vi "Control.vi"() -> ()   [LabVIEW 2020]
uses:
  proceso1.vi
  proceso2.vi
  proceso3.vi
  proceso4.vi
  proceso5.vi
  proceso6.vi
panel:
  in  "Numeric 14":dbl
  in  "Numeric 13":dbl
  in  "Numeric 12":dbl
  in  "Numeric 11":dbl
  in  "Numeric 10":dbl
  out "Boolean":bool
  in  "Numeric 9":dbl
  in  "Numeric 8":dbl
  in  "Numeric 7":dbl
  in  "Numeric 6":dbl
  in  "Numeric 5":dbl
  in  "Numeric 4":dbl
  in  "Numeric 3":dbl
  in  "Numeric 2":dbl
  out "s? t:f":dbl
  in  "Numeric":dbl
types:
  T1 = typedef "Semaphore RefNum" = refnum<k1>
  T2 = cluster{"final_linea":bool, "vent 1":bool, "vent 2":bool, "vent 3":bool, "mov caja 2 horizontal":i32, "llenado caja 2":u8, "pos_inicial_horizontal":dbl, " pos_final_horizontal":dbl, "contador":dbl, "mov caja 2  vertical":i32, "pos_inicial_vertical":dbl, " pos_final_vertical":dbl}
  T3 = cluster{"sensor_refrigerador":bool, "temperatura":dbl, "tuberia 5":u8, "tuberia 6":u8}
  T4 = cluster{"sensor_intercambiador":bool, "sensor_caldera":bool, "sensor_bomba_2 ":bool, "tuberia 2":u8, "tuberia 3":u8, "tuberia 4":u8, "temperatura":dbl}
  T5 = cluster{"sensor_bomba_1":bool, "tanque in":u8, " tuberia 1":u8}
  T6 = cluster{"sensor_caja":bool, "vent 1":bool, "vent 2":bool, "vent 3":bool, "pos_inicial":dbl, "pos_final":dbl, "mov_caja 1":i32}
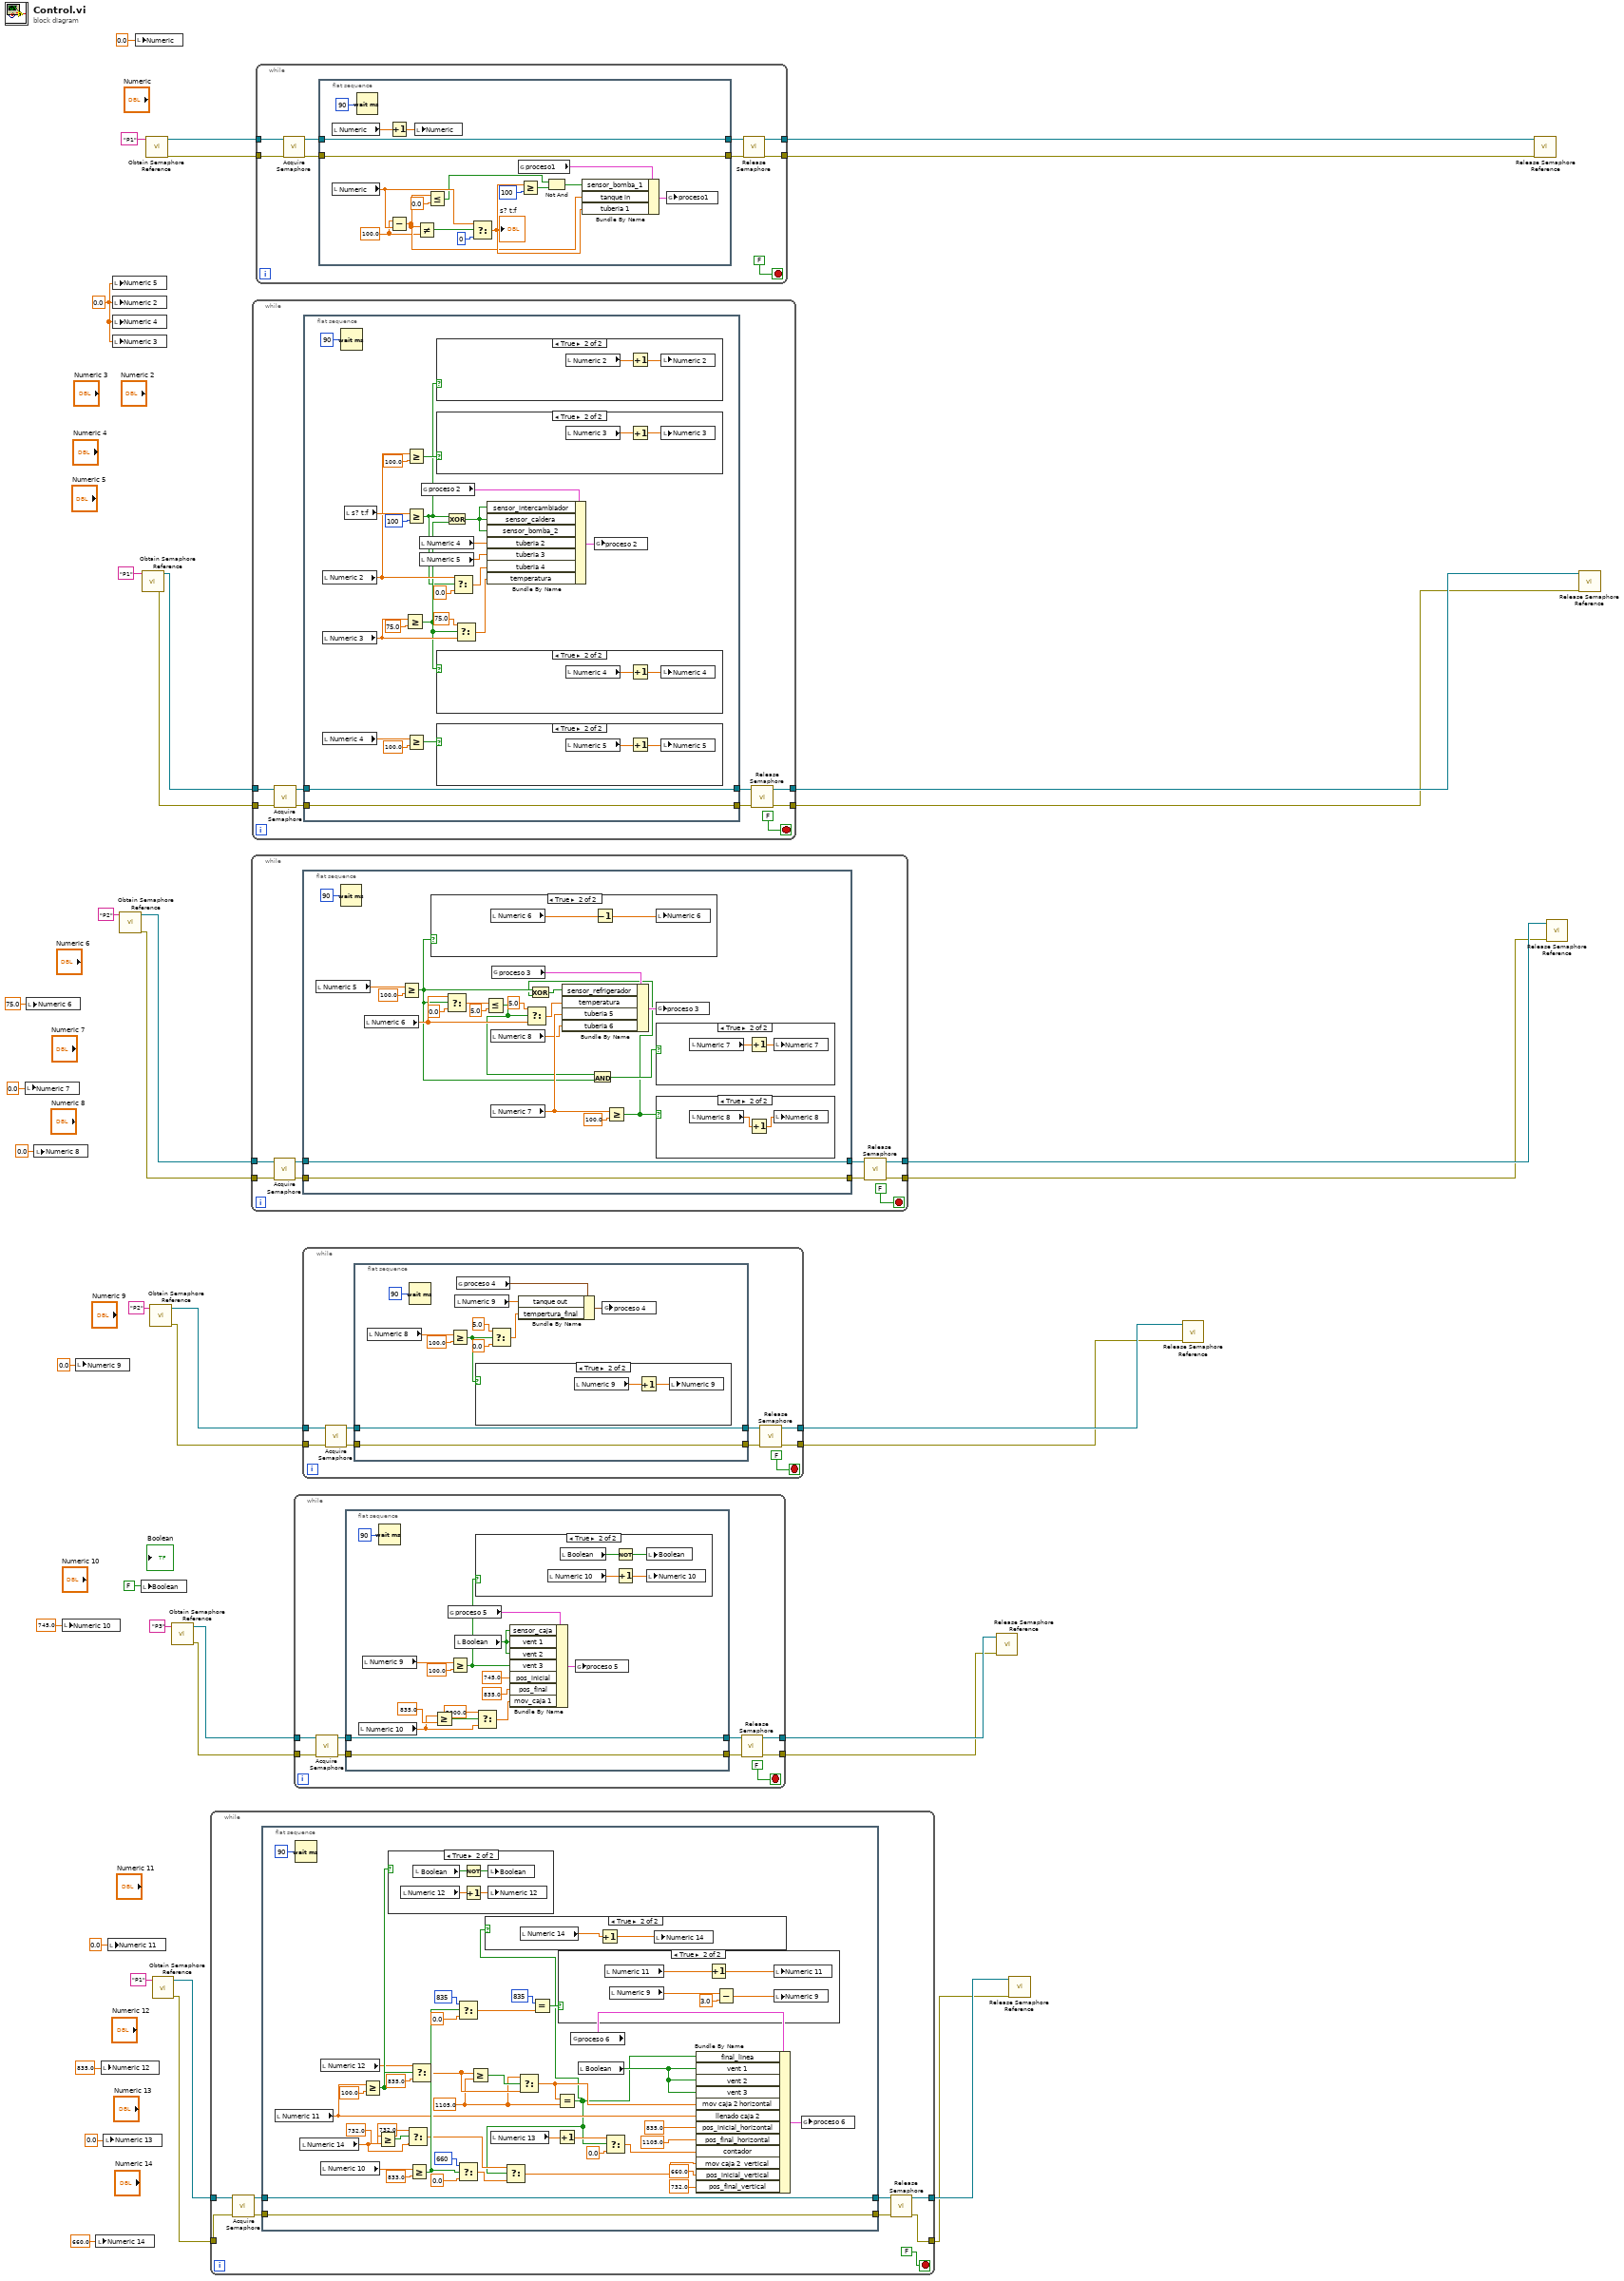
[diagram p0: block diagram]
diagram:
  w31 = 0.0 ("Numeric 2")
  n1 = local write "Numeric 7"(0.0 ("Numeric 7")) -> ()
  n2 = local write "Numeric 6"(75.0 ("Numeric 6")) -> ()
  n3 = local write "Numeric 8"(0.0 ("Numeric 8")) -> ()
  n4 = local write "Numeric 10"(745.0 ("Numeric 10")) -> ()
  n5 = local write "Numeric 9"(0.0 ("Numeric 9")) -> ()
  n6 = local write "Numeric 14"(660.0 ("Numeric 14")) -> ()
  n7 = local write "Numeric 12"(835.0 ("Numeric 12")) -> ()
  n8 = local write "Numeric 13"(0.0 ("Numeric 13")) -> ()
  n9 = local write "Numeric 11"(0.0 ("Numeric 11")) -> ()
  n10 = local write "Numeric 5"(w31) -> ()
  n11 = local write "Numeric 2"(w31) -> ()
  n12 = local write "Numeric 4"(w31) -> ()
  n13 = local write "Numeric 3"(w31) -> ()
  n14 = call <vilib>:"Obtain Semaphore Reference.vi"("name (unnamed)"="P2") -> ("error out"=w29:errorcluster, "semaphore"=w30:T1)  [unwired: 4 in, 1 out]
  n15 = local write "Numeric"(0.0 ("Numeric")) -> ()
  n16 = local write "Boolean"(FALSE ("Boolean")) -> ()
  n17 = call <vilib>:"Obtain Semaphore Reference.vi"("name (unnamed)"="P1") -> ("error out"=w33:errorcluster, "semaphore"=w32:T1)  [unwired: 4 in, 1 out]
  n18 = call <vilib>:"Obtain Semaphore Reference.vi"("name (unnamed)"="P1") -> ("error out"=w35:errorcluster, "semaphore"=w34:T1)  [unwired: 4 in, 1 out]
  n19 = call <vilib>:"Obtain Semaphore Reference.vi"("name (unnamed)"="P2") -> ("error out"=w21:errorcluster, "semaphore"=w22:T1)  [unwired: 4 in, 1 out]
  n20 = call <vilib>:"Obtain Semaphore Reference.vi"("name (unnamed)"="P1") -> ("error out"=w9:errorcluster, "semaphore"=w10:T1)  [unwired: 4 in, 1 out]
  n21 = call <vilib>:"Obtain Semaphore Reference.vi"("name (unnamed)"="P3") -> ("error out"=w16:errorcluster, "semaphore"=w17:T1)  [unwired: 4 in, 1 out]
  n22 = while {
    tunnel: w10 -> [w50]
    tunnel: w9 -> [w49]
    tunnel: [w44] -> w8
    tunnel: [w43] -> w7
    stop <- FALSE stop-if-true
    n23 = call <vilib>:"Acquire Semaphore.vi"("error in (no error)"=w49, "semaphore"=w50) -> ("error out"=w46:errorcluster, "semaphore out"=w48:T1)  [unwired: 3 in, 1 out]
    n24 = flat-sequence {
      tunnel: w48 -> [w81]
      tunnel: [w81] -> w47
      tunnel: w46 -> [w89]
      tunnel: [w89] -> w45
      frame #0 {
        w64 = 1105.0 ("y")
        n25 = local read "Numeric 11"() -> (w73:dbl)
        n26 = Wait (ms)(milliseconds to wait=u32 90) -> ()  [unwired: 1 out]
        n27 = local read "Numeric 14"() -> (w56:dbl)
        n28 = local read "Numeric 12"() -> (w68:dbl)
        n29 = local read "Numeric 10"() -> (w86:dbl)
        n30 = Greater Or Equal?(x=w73, y=100.0) -> (x >= y?=w69:bool)
        n31 = Greater Or Equal?(x=w56, y=732.0) -> (x >= y?=w58:bool)
        n32 = case shown="True" w69 {
          frame False {
          }
          frame True {
            n33 = local read "Numeric 12"() -> (w98:dbl)
            n34 = local read "Boolean"() -> (w95:bool)
            n35 = Not(x=w95) -> (.not. x?=w96:bool)
            n36 = Increment(x=w98) -> (x+1=w97:dbl)
            n37 = local write "Boolean"(w96) -> ()
            n38 = local write "Numeric 12"(w97) -> ()
          }
        }
        n39 = Select(t=732.0, s=w58, f=w56) -> (s? t:f=w55:dbl)
        n40 = Greater Or Equal?(x=w86, y=833.0) -> (x >= y?=w83:bool)
        n41 = Select(t=w68, s=w69, f=835.0) -> (s? t:f=w66:dbl)
        n42 = Select(t=835 ("mov caja 2 horizontal"), s=w83, f=0.0) -> (s? t:f=w71:dbl)
        n43 = Select(t=660 ("mov caja 2  vertical"), s=w83, f=0.0) -> (s? t:f=w54:dbl)
        n44 = Greater Or Equal?(x=w66, y=w64) -> (x >= y?=w67:bool)
        n45 = local read "Numeric 13"() -> (w63:dbl)
        n46 = Select(t=w64, s=w67, f=w66) -> (s? t:f=w65:dbl)
        n47 = Equal?(x=835, y=w71) -> (x = y?=w75:bool)
        n48 = Equal?(x=w65, y=w64) -> (x = y?=w52:bool)
        n49 = case shown="True" w52 {
          frame False {
          }
          frame True {
            n50 = local read "Numeric 14"() -> (w93:dbl)
            n51 = Increment(x=w93) -> (x+1=w94:dbl)
            n52 = local write "Numeric 14"(w94) -> ()
          }
        }
        n53 = Select(t=w55, s=w52, f=w54) -> (s? t:f=w53:dbl)
        n54 = Increment(x=w63) -> (x+1=w62:dbl)
        n55 = case shown="True" w75 {
          frame False {
          }
          frame True {
            n56 = local read "Numeric 11"() -> (w103:dbl)
            n57 = local read "Numeric 9"() -> (w101:dbl)
            n58 = Increment(x=w103) -> (x+1=w102:dbl)
            n59 = Subtract(x=w101, y=3.0) -> (x-y=w100:dbl)
            n60 = local write "Numeric 11"(w102) -> ()
            n61 = local write "Numeric 9"(w100) -> ()
          }
        }
        n62 = global read "proceso6.vi" "proceso 6"() -> (w92:T2)
        n63 = local read "Boolean"() -> (w90:bool)
        n64 = Select(t=w62, s=w52, f=0.0) -> (s? t:f=w60:dbl)
        n65 = Bundle By Name(cluster=w92, "final_linea"=w52, "vent 1"=w90, "vent 2"=w90, "vent 3"=w90, "mov caja 2 horizontal"=w65, "llenado caja 2"=w73, "pos_inicial_horizontal"=835.0, "pos_final_horizontal"=1105.0, "contador"=w60, "mov caja 2  vertical"=w53, "pos_inicial_vertical"=660.0, "pos_final_vertical"=732.0) -> (w91:T2)
        n66 = global write "proceso6.vi" "proceso 6"(w91) -> ()
      }
    }
    n67 = call <vilib>:"Release Semaphore.vi"("error in (no error)"=w45, "semaphore"=w47) -> ("error out"=w43:errorcluster, "semaphore out"=w44:T1)  [unwired: 4 in]
  }
  n68 = while {
    tunnel: w30 -> [w111]
    tunnel: w29 -> [w110]
    tunnel: [w105] -> w28
    tunnel: [w104] -> w27
    stop <- FALSE stop-if-true
    n69 = call <vilib>:"Acquire Semaphore.vi"("error in (no error)"=w110, "semaphore"=w111) -> ("error out"=w108:errorcluster, "semaphore out"=w109:T1)  [unwired: 3 in, 1 out]
    n70 = flat-sequence {
      tunnel: w109 -> [w129]
      tunnel: w108 -> [w128]
      tunnel: [w129] -> w107
      tunnel: [w128] -> w106
      frame #0 {
        n71 = local read "Numeric 5"() -> (w131:dbl)
        n72 = Wait (ms)(milliseconds to wait=u32 90) -> ()  [unwired: 1 out]
        n73 = local read "Numeric 6"() -> (w122:dbl)
        n74 = Greater Or Equal?(x=w131, y=100.0) -> (x >= y?=w115:bool)
        n75 = case shown="True" w115 {
          frame False {
          }
          frame True {
            n76 = local read "Numeric 6"() -> (w139:dbl)
            n77 = Decrement(x=w139) -> (x-1=w138:dbl)
            n78 = local write "Numeric 6"(w138) -> ()
          }
        }
        n79 = Select(t=w122, s=w115, f=0.0) -> (s? t:f=w125:dbl)
        n80 = Less Or Equal?(x=w125, y=5.0) -> (x <= y?=w117:bool)
        n81 = local read "Numeric 8"() -> (w119:dbl)
        n82 = local read "Numeric 7"() -> (w120:dbl)
        n83 = global read "proceso3.vi" "proceso 3"() -> (w133:T3)
        n84 = Select(t=5.0, s=w117, f=w122) -> (s? t:f=w118:dbl)
        n85 = And(x=w117, y=w115) -> (x .and. y?=w116:bool)
        n86 = Greater Or Equal?(x=w120, y=100.0) -> (x >= y?=w114:bool)
        n87 = Exclusive Or(1:w114, 2:w115) -> (0:w113:bool)
        n88 = Bundle By Name(cluster=w133, "sensor_refrigerador"=w113, "temperatura"=w118, "tuberia 5"=w120, "tuberia 6"=w119) -> (w132:T3)
        n89 = global write "proceso3.vi" "proceso 3"(w132) -> ()
        n90 = case shown="True" w116 {
          frame False {
          }
          frame True {
            n91 = local read "Numeric 7"() -> (w137:dbl)
            n92 = Increment(x=w137) -> (x+1=w136:dbl)
            n93 = local write "Numeric 7"(w136) -> ()
          }
        }
        n94 = case shown="True" w114 {
          frame False {
          }
          frame True {
            n95 = local read "Numeric 8"() -> (w135:dbl)
            n96 = Increment(x=w135) -> (x+1=w134:dbl)
            n97 = local write "Numeric 8"(w134) -> ()
          }
        }
      }
    }
    n98 = call <vilib>:"Release Semaphore.vi"("error in (no error)"=w106, "semaphore"=w107) -> ("error out"=w104:errorcluster, "semaphore out"=w105:T1)  [unwired: 4 in]
  }
  n99 = while {
    tunnel: [w147] -> w40
    tunnel: [w146] -> w39
    tunnel: w33 -> [w145]
    tunnel: w32 -> [w144]
    stop <- FALSE stop-if-true
    n100 = call <vilib>:"Acquire Semaphore.vi"("error in (no error)"=w145, "semaphore"=w144) -> ("error out"=w142:errorcluster, "semaphore out"=w143:T1)  [unwired: 3 in, 1 out]
    n101 = flat-sequence {
      tunnel: w143 -> [w166]
      tunnel: w142 -> [w165]
      tunnel: [w166] -> w141
      tunnel: [w165] -> w140
      frame #0 {
        n102 = local read "Numeric 2"() -> (w159:dbl)
        n103 = local read "Numeric 3"() -> (w160:dbl)
        n104 = local read "Numeric 4"() -> (w155:dbl)
        n105 = Wait (ms)(milliseconds to wait=u32 90) -> ()  [unwired: 1 out]
        n106 = local read "s? t:f"() -> (w170:dbl)
        n107 = Greater Or Equal?(x=w160, y=75.0) -> (x >= y?=w151:bool)
        n108 = Greater Or Equal?(x=w159, y=100.0 ("x")) -> (x >= y?=w157:bool)
        n109 = Greater Or Equal?(x=w170, y=100) -> (x >= y?=w150:bool)
        n110 = Greater Or Equal?(x=w155, y=100.0) -> (x >= y?=w156:bool)
        n111 = local read "Numeric 4"() -> (w153:dbl)
        n112 = local read "Numeric 5"() -> (w152:dbl)
        n113 = global read "proceso2.vi" "proceso 2"() -> (w171:T4)
        n114 = case shown="True" w150 {
          frame False {
          }
          frame True {
            n115 = local read "Numeric 2"() -> (w179:dbl)
            n116 = Increment(x=w179) -> (x+1=w180:dbl)
            n117 = local write "Numeric 2"(w180) -> ()
          }
        }
        n118 = case shown="True" w157 {
          frame False {
          }
          frame True {
            n119 = local read "Numeric 3"() -> (w177:dbl)
            n120 = Increment(x=w177) -> (x+1=w178:dbl)
            n121 = local write "Numeric 3"(w178) -> ()
          }
        }
        n122 = case shown="True" w151 {
          frame False {
          }
          frame True {
            n123 = local read "Numeric 4"() -> (w176:dbl)
            n124 = Increment(x=w176) -> (x+1=w175:dbl)
            n125 = local write "Numeric 4"(w175) -> ()
          }
        }
        n126 = case shown="True" w156 {
          frame False {
          }
          frame True {
            n127 = local read "Numeric 5"() -> (w174:dbl)
            n128 = Increment(x=w174) -> (x+1=w173:dbl)
            n129 = local write "Numeric 5"(w173) -> ()
          }
        }
        n130 = Exclusive Or(1:w151, 2:w150) -> (0:w149:bool)
        n131 = Select(t=w159, s=w150, f=0.0) -> (s? t:f=w167:dbl)
        n132 = Select(t=75.0, s=w151, f=w160) -> (s? t:f=w162:dbl)
        n133 = Bundle By Name(cluster=w171, "sensor_intercambiador"=w149, "sensor_caldera"=w149, "sensor_bomba_2"=w149, "tuberia 2"=w153, "tuberia 3"=w152, "tuberia 4"=w167, "temperatura"=w162) -> (w172:T4)
        n134 = global write "proceso2.vi" "proceso 2"(w172) -> ()
      }
    }
    n135 = call <vilib>:"Release Semaphore.vi"("error in (no error)"=w140, "semaphore"=w141) -> ("error out"=w146:errorcluster, "semaphore out"=w147:T1)  [unwired: 4 in]
  }
  n136 = while {
    tunnel: [w188] -> w37
    tunnel: [w187] -> w36
    tunnel: w35 -> [w184]
    tunnel: w34 -> [w183]
    stop <- FALSE stop-if-true
    n137 = call <vilib>:"Acquire Semaphore.vi"("error in (no error)"=w184, "semaphore"=w183) -> ("error out"=w182:errorcluster, "semaphore out"=w181:T1)  [unwired: 3 in, 1 out]
    n138 = flat-sequence {
      tunnel: w181 -> [w191]
      tunnel: [w191] -> w186
      tunnel: w182 -> [w190]
      tunnel: [w190] -> w185
      frame #0 {
        w192 = 100.0 ("x")
        n139 = local read "Numeric"() -> (w205:dbl)
        n140 = local read "Numeric"() -> (w207:dbl)
        n141 = Wait (ms)(milliseconds to wait=u32 90) -> ()  [unwired: 1 out]
        n142 = Increment(x=w205) -> (x+1=w206:dbl)
        n143 = Subtract(x=w192, y=w207) -> (x-y=w200:dbl)
        n144 = local write "Numeric"(w206) -> ()
        n145 = Not Equal?(x=w200, y=w192) -> (x != y?=w199:bool)
        n146 = Less Or Equal?(x=w200, y=0.0) -> (x <= y?=w201:bool)
        n147 = Select(t=w207, s=w199, f=0) -> (s? t:f=w204:dbl)
        "s? t:f" <- w204
        n148 = global read "proceso1.vi" "proceso1"() -> (w197:T5)
        n149 = Greater Or Equal?(x=w204, y=100) -> (x >= y?=w202:bool)
        n150 = Not And(1:w202, 2:w201) -> (0:w203:bool)
        n151 = Bundle By Name(cluster=w197, "sensor_bomba_1"=w203, "tanque in"=w200, "tuberia 1"=w204) -> (w198:T5)
        n152 = global write "proceso1.vi" "proceso1"(w198) -> ()
      }
    }
    n153 = call <vilib>:"Release Semaphore.vi"("error in (no error)"=w185, "semaphore"=w186) -> ("error out"=w188:errorcluster, "semaphore out"=w187:T1)  [unwired: 4 in]
  }
  n154 = while {
    tunnel: w17 -> [w215]
    tunnel: w16 -> [w214]
    tunnel: [w209] -> w15
    tunnel: [w208] -> w14
    stop <- FALSE stop-if-true
    n155 = call <vilib>:"Acquire Semaphore.vi"("error in (no error)"=w214, "semaphore"=w215) -> ("error out"=w212:errorcluster, "semaphore out"=w213:T1)  [unwired: 3 in, 1 out]
    n156 = flat-sequence {
      tunnel: w213 -> [w228]
      tunnel: w212 -> [w227]
      tunnel: [w228] -> w211
      tunnel: [w227] -> w210
      frame #0 {
        n157 = local read "Numeric 10"() -> (w219:dbl)
        n158 = local read "Numeric 9"() -> (w229:dbl)
        n159 = Wait (ms)(milliseconds to wait=u32 90) -> ()  [unwired: 1 out]
        n160 = Greater Or Equal?(x=w219, y=835.0) -> (x >= y?=w221:bool)
        n161 = global read "proceso5.vi" "proceso 5"() -> (w232:T6)
        n162 = Greater Or Equal?(x=w229, y=100.0) -> (x >= y?=w225:bool)
        n163 = local read "Boolean"() -> (w224:bool)
        n164 = case shown="True" w225 {
          frame False {
          }
          frame True {
            n165 = local read "Numeric 10"() -> (w233:dbl)
            n166 = local read "Boolean"() -> (w235:bool)
            n167 = Not(x=w235) -> (.not. x?=w236:bool)
            n168 = Increment(x=w233) -> (x+1=w234:dbl)
            n169 = local write "Boolean"(w236) -> ()
            n170 = local write "Numeric 10"(w234) -> ()
          }
        }
        n171 = Select(t=2000.0, s=w221, f=w219) -> (s? t:f=w218:dbl)
        n172 = Bundle By Name(cluster=w232, "sensor_caja"=w224, "vent 1"=w224, "vent 2"=w224, "vent 3"=w225, "pos_inicial"=745.0, "pos_final"=835.0, "mov_caja 1"=w218) -> (w231:T6)
        n173 = global write "proceso5.vi" "proceso 5"(w231) -> ()
      }
    }
    n174 = call <vilib>:"Release Semaphore.vi"("error in (no error)"=w210, "semaphore"=w211) -> ("error out"=w208:errorcluster, "semaphore out"=w209:T1)  [unwired: 4 in]
  }
  n175 = while {
    tunnel: w22 -> [w244]
    tunnel: w21 -> [w243]
    tunnel: [w238] -> w20
    tunnel: [w237] -> w19
    stop <- FALSE stop-if-true
    n176 = call <vilib>:"Acquire Semaphore.vi"("error in (no error)"=w243, "semaphore"=w244) -> ("error out"=w241:errorcluster, "semaphore out"=w242:T1)  [unwired: 3 in, 1 out]
    n177 = flat-sequence {
      tunnel: w242 -> [w255]
      tunnel: w241 -> [w254]
      tunnel: [w255] -> w240
      tunnel: [w254] -> w239
      frame #0 {
        n178 = local read "Numeric 8"() -> (w253:dbl)
        n179 = Wait (ms)(milliseconds to wait=u32 90) -> ()  [unwired: 1 out]
        n180 = Greater Or Equal?(x=w253, y=100.0) -> (x >= y?=w250:bool)
        n181 = local read "Numeric 9"() -> (w251:dbl)
        n182 = global read "proceso4.vi" "proceso 4"() -> (w257:cluster{"tanque out":u8, "tempertura_final":dbl})
        n183 = case shown="True" w250 {
          frame False {
          }
          frame True {
            n184 = local read "Numeric 9"() -> (w259:dbl)
            n185 = Increment(x=w259) -> (x+1=w258:dbl)
            n186 = local write "Numeric 9"(w258) -> ()
          }
        }
        n187 = Select(t=5.0, s=w250, f=0.0) -> (s? t:f=w249:dbl)
        n188 = Bundle By Name(cluster=w257, "tanque out"=w251, "tempertura_final"=w249) -> (w256:cluster{"tanque out":u8, "tempertura_final":dbl})
        n189 = global write "proceso4.vi" "proceso 4"(w256) -> ()
      }
    }
    n190 = call <vilib>:"Release Semaphore.vi"("error in (no error)"=w239, "semaphore"=w240) -> ("error out"=w237:errorcluster, "semaphore out"=w238:T1)  [unwired: 4 in]
  }
  n191 = call <vilib>:"Release Semaphore Reference.vi"("error in (no error)"=w14, "semaphore"=w15) -> ()  [unwired: 8 in, 2 out]
  n192 = call <vilib>:"Release Semaphore Reference.vi"("error in (no error)"=w7, "semaphore"=w8) -> ()  [unwired: 8 in, 2 out]
  n193 = call <vilib>:"Release Semaphore Reference.vi"("error in (no error)"=w19, "semaphore"=w20) -> ()  [unwired: 8 in, 2 out]
  n194 = call <vilib>:"Release Semaphore Reference.vi"("error in (no error)"=w37, "semaphore"=w36) -> ()  [unwired: 8 in, 2 out]
  n195 = call <vilib>:"Release Semaphore Reference.vi"("error in (no error)"=w27, "semaphore"=w28) -> ()  [unwired: 8 in, 2 out]
  n196 = call <vilib>:"Release Semaphore Reference.vi"("error in (no error)"=w39, "semaphore"=w40) -> ()  [unwired: 8 in, 2 out]
